vi "Abort Logger.vi"(8 "Error In":errorcluster, 11 "TDMS Log In":refnum<class "TDMS Logger.lvclass">) -> (0 "Error Out":errorcluster)   [LabVIEW 2014, in "TDMS Logger.lvlib" / "TDMS Logger.lvclass"]
doc: "This VI will abort the data logger. All data that was not saved and is still in the data logger queue will be discarded.\n\nMaximum time spent in this VI waiting for the asynchronous logging loop to abort is 50ms.\n<b>If that time is not enough then the TDMS file reference might remain open.</b>\n\nTo be sure and safe while stopping the logging please use the <b>Log Rest and Release</b> method."
uses:
  TDMS Logger.lvclass
  _Typedefs/Log Message.ctl
  _Typedefs/Log Action.ctl
  _Typedefs/Data Type.ctl
  TDMS Logger.lvclass/TDMS Logger.ctl
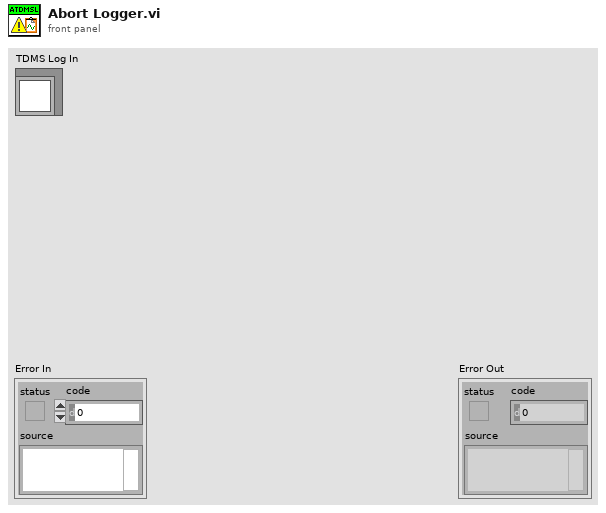
[diagram p1: front panel]
types:
  T1 = typedef "TDMS Logger.lvlib/TDMS Logger.lvclass/Log Action.ctl" = enum16{"Handle Old Files", "Status Update", "Stop", "Log Data", "Initialize"}
  T2 = typedef "TDMS Logger.lvlib/TDMS Logger.lvclass/Log Message.ctl" = cluster{"Log Action":T1, "Variant":variant, "Data Type":T3, "Group Name":string, "Channels Names":string[]}
  T3 = typedef "TDMS Logger.lvlib/TDMS Logger.lvclass/Data Type.ctl" = enum16{"I16", "I8", "String", "U16", "U8", "Waveform", "Double", "Single"}
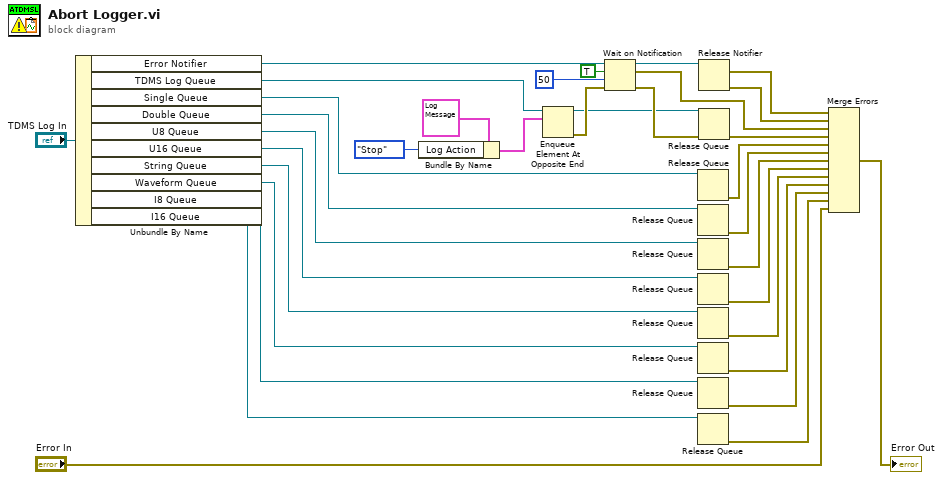
[diagram p0: block diagram]
diagram:
  n1 = Unbundle By Name("TDMS Log In") -> ("Error Notifier"=w33:refnum<notifier>, "TDMS Log Queue"=w5:refnum<queue>, "Single Queue"=w18:refnum<queue>, "Double Queue"=w17:refnum<queue>, "U8 Queue"=w16:refnum<queue>, "U16 Queue"=w15:refnum<queue>, "String Queue"=w14:refnum<queue>, "Waveform Queue"=w13:refnum<queue>, "I8 Queue"=w2:refnum<queue>, "I16 Queue"=w1:refnum<queue>)
  n2 = Bundle By Name(cluster=T2 {"Log Action"=enum."Stop", "Variant"=variant, "Data Type"=enum."String", "Group Name"="", "Channels Names"=[]} ("element"), "Log Action"=Log_Action."Stop") -> (w27:T2)
  n3 = Enqueue Element At Opposite End(queue=w5, element=w27) -> (queue out=w20:refnum<queue>, error out=w22:errorcluster)  [unwired: 2 in, 1 out]
  n4 = Wait on Notification(notifier=w33, ignore previous (F)=TRUE, timeout in ms (-1)=50, error in (no error)=w22) -> (notifier out=w25:refnum<notifier>, notification=w19:errorcluster, error out=w21:errorcluster)  [unwired: 1 out]
  n5 = Release Queue(queue=w18) -> (error out=w12:errorcluster)  [unwired: 2 in, 2 out]
  n6 = Release Queue(queue=w17) -> (error out=w11:errorcluster)  [unwired: 2 in, 2 out]
  n7 = Release Queue(queue=w16) -> (error out=w10:errorcluster)  [unwired: 2 in, 2 out]
  n8 = Release Queue(queue=w15) -> (error out=w9:errorcluster)  [unwired: 2 in, 2 out]
  n9 = Release Queue(queue=w14) -> (error out=w8:errorcluster)  [unwired: 2 in, 2 out]
  n10 = Release Queue(queue=w13) -> (error out=w7:errorcluster)  [unwired: 2 in, 2 out]
  n11 = Release Queue(queue=w2) -> (error out=w4:errorcluster)  [unwired: 2 in, 2 out]
  n12 = Release Queue(queue=w1) -> (error out=w3:errorcluster)  [unwired: 2 in, 2 out]
  n13 = Release Notifier(notifier=w25) -> (last notification=w30:errorcluster, error out=w31:errorcluster)  [unwired: 2 in, 1 out]
  n14 = Release Queue(queue=w20, error in (no error)=w21) -> (error out=w32:errorcluster)  [unwired: 1 in, 2 out]
  n15 = Merge Errors(w30, w31, w19, w32, w12, w11, w10, w9, w8, w7, w4, w3, "Error In") -> (→"Error Out":errorcluster)
